vi "Test.vi"() -> ()   [LabVIEW 2012, in "DimActorDemo.lvlib"]
doc: "To be used for testing only."
uses:
  DimActorDemo.lvlib
  DIMDemoClient/DIMDemoClient.lvclass
  DIMDemoServer/DIMDemoServer.lvclass
  DIMActor/DIMActor/DIMActor.lvclass/DIMActor.ctl
  DIMDemoClient/DIMDemoClient.lvclass/DIMDemoClient.ctl
  <vilib>/ActorFramework/Message Queue/Message Queue.lvclass/Message Queue.ctl
  <vilib>/ActorFramework/Message Enqueuer/Message Enqueuer.lvclass/Message Enqueuer.ctl
  <vilib>/ActorFramework/Message Enqueuer/Enqueue.vi
  <vilib>/ActorFramework/Message Priority Queue/Priority Enqueue.vi
  <vilib>/ActorFramework/Stop Msg/Stop Msg.lvclass
  <vilib>/ActorFramework/Actor/Actor.lvclass
  <vilib>/ActorFramework/Message Queue/Message Queue.lvclass
  DIMActor/DIMActor/DIMActor.lvclass
panel:
  out "Error Out":errorcluster
  in  "Stop Button":bool
  # "LVDimInterface.lvlib:LVDimInterface.dim_operate.vi\nneed to be started first!"
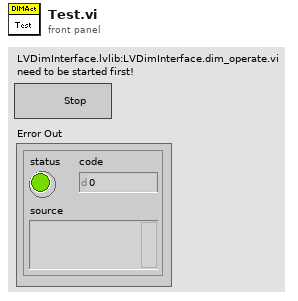
[diagram p1: front panel]
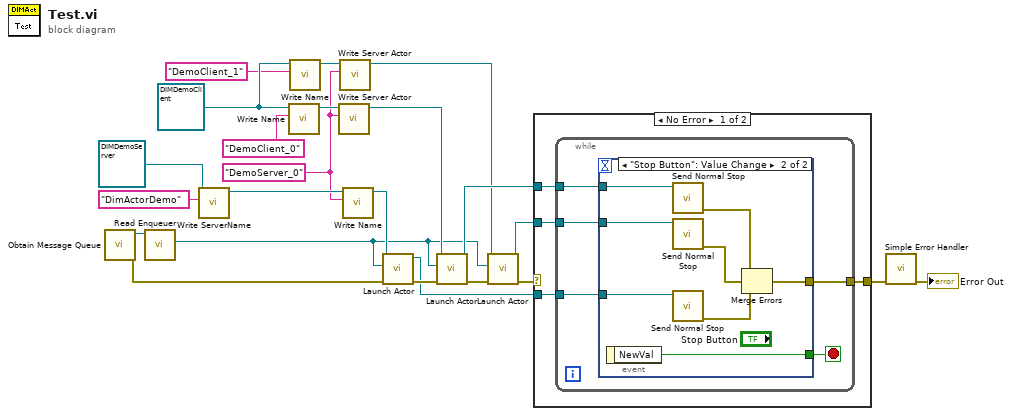
[diagram p0: block diagram]
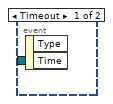
[diagram p2: hidden frame]
diagram:
  w7 = "DemoServer_0" ("Name")
  w8 = refnum<class "DIMDemoClient.lvclass"> refnum ("DimActorDemo.lvlib:DIMDemoClient.lvclass")
  n1 = call <vilib>:"Obtain Message Queue.vi"() -> ("error out"=w19:errorcluster, "Message Queue"=w23:refnum<class "Message Queue.lvclass">)  [unwired: 10 in]
  n2 = call <vilib>:"Read Enqueuer.vi"("Message Queue"=w23) -> ("Message Enqueuer"=w2:refnum<class "Message Enqueuer.lvclass">)  [unwired: 10 in]
  n3 = call "Write ServerName.vi"("ServerName"="DimActorDemo", "DIMActor in"=refnum<class "DIMDemoServer.lvclass"> refnum ("DimActorDemo.lvlib:DIMDemoServer.lvclass")) -> ("DIMActor out"=w14:refnum<class "DIMDemoServer.lvclass">)  [unwired: 8 in, 1 out]
  n4 = call "Write Name.vi"("Name"="DemoClient_0", "DIMActor in"=w8) -> ("DIMActor out"=w11:refnum<class "DIMDemoClient.lvclass">)  [unwired: 8 in, 1 out]
  n5 = call "Write Name.vi"("Name"="DemoClient_1", "DIMActor in"=w8) -> ("DIMActor out"=w9:refnum<class "DIMDemoClient.lvclass">)  [unwired: 8 in, 1 out]
  n6 = call "Write Server Actor.vi"("Server Actor"=w7, "DIMDemoClient in"=w11) -> ("DIMDemoClient out"=w10:refnum<class "DIMDemoClient.lvclass">)  [unwired: 8 in, 1 out]
  n7 = call "Write Server Actor.vi"("Server Actor"=w7, "DIMDemoClient in"=w9) -> ("DIMDemoClient out"=w3:refnum<class "DIMDemoClient.lvclass">)  [unwired: 8 in, 1 out]
  n8 = call "Write Name.vi"("Name"=w7, "DIMActor in"=w14) -> ("DIMActor out"=w13:refnum<class "DIMDemoServer.lvclass">)  [unwired: 8 in, 1 out]
  n9 = call <vilib>:"Launch Actor.vi"("error in (no error)"=w19, "Actor-to-Caller Enqueuer"=w2, "Actor"=w13) -> ("error out"=w18:errorcluster, "Caller-To-Actor Enqueuer"=w17:refnum<class "Message Enqueuer.lvclass">)  [unwired: 7 in]
  n10 = call <vilib>:"Launch Actor.vi"("error in (no error)"=w18, "Actor-to-Caller Enqueuer"=w2, "Actor"=w10) -> ("error out"=w5:errorcluster, "Caller-To-Actor Enqueuer"=w22:refnum<class "Message Enqueuer.lvclass">)  [unwired: 7 in]
  n11 = call <vilib>:"Launch Actor.vi"("error in (no error)"=w5, "Actor-to-Caller Enqueuer"=w2, "Actor"=w3) -> ("error out"=w4:errorcluster, "Caller-To-Actor Enqueuer"=w1:refnum<class "Message Enqueuer.lvclass">)  [unwired: 7 in]
  n12 = case shown="No Error" w4 {
    selector: w4 -> [_ w41]
    tunnel: w22 -> [w27 _]
    tunnel: [w24 w41] -> w21
    tunnel: w17 -> [w26 _]
    tunnel: w1 -> [w25 _]
    frame No Error {
      n13 = while {
        tunnel: w27 -> [w31]
        tunnel: w26 -> [w30]
        tunnel: w25 -> [w29]
        tunnel: [w28] -> w24
        stop <- w32 stop-if-true
        n14 = event shown="[1] \"Stop Button\": Value Change" {
          selector: _ -> [_ _]
          dyn-events: _ -> [_ _]
          timeout: _ -> [_ _]
          tunnel: [_ w40] -> w32
          tunnel: w31 -> [_ w39]
          tunnel: w30 -> [_ w38]
          tunnel: w29 -> [_ w37]
          tunnel: [_ w33] -> w28
          event Timeout {
            n15 = event-data() -> ()  [unwired: 1 in, 2 out]
          }
          event "Stop Button": Value Change {
            n16 = event-data() -> ("NewVal"=w40:bool)  [unwired: 1 in]
            n17 = call <vilib>:"Send Normal Stop.vi"("Message Enqueuer"=w39) -> ("error out"=w36:errorcluster)  [unwired: 10 in]
            n18 = call <vilib>:"Send Normal Stop.vi"("Message Enqueuer"=w37) -> ("error out"=w35:errorcluster)  [unwired: 10 in]
            n19 = call <vilib>:"Send Normal Stop.vi"("Message Enqueuer"=w38) -> ("error out"=w34:errorcluster)  [unwired: 10 in]
            n20 = Merge Errors(w36, w35, w34) -> (w33:errorcluster)
          }
        }
      }
    }
    frame Error {
    }
  }
  n21 = call <vilib>:"Simple Error Handler.vi"("error in (no error)"=w21) -> ("error out"=→"Error Out":errorcluster)  [unwired: 4 in, 4 out]
